vi "Generate Hologram.vi"(0 "x":sgl[](array[numeric]), 1 "y":sgl[](array[numeric]), 2 "z":sgl[](array[numeric]), 3 "spot_intensities":sgl[](array[numeric]) min=1, 4 "CUDA/SLM error in":errorcluster, 8 "path in":path, 9 "N_iterations":i32, 10 "method":i32, 12 "CGH in":u8[][](array[numeric])=array512x512[262144 elements]) -> (18 "path out":path, 20 "return":i32, 24 "CGH out":u8[][](array[numeric]), 25 "weights":sgl[][](graph)=[[0.32087266, 0.30867794, 0.31952837, 0.32111803, 0.32117248, 0.3210771, 0.32099402, 0.32094038, 0.32090643, 0.32088554], [0.32087216, 0.30864686, 0.31954217, 0.32109785, 0.3211845, 0.32108435, 0.32099703, 0.32094118, 0.3209064, 0.32088524], [0.32087475, 0.30863738, 0.3195775, 0.3210921, 0.32118624, 0.3210818, 0.32099742, 0.32094282, 0.32090908, 0.32088798], [0.3208743, 0.3086348, 0.31957102, 0.3210825, 0.3211723, 0.32108226, 0.32100248, 0.3209465, 0.3209109, 0.3208884], [0.32082918, 0.33360976, 0.32222247, 0.3205971, 0.32050273, 0.32060897, 0.32069725, 0.32075626, 0.3207928, 0.3208153], [0.3208285, 0.33361444, 0.32216293, 0.32054555, 0.32047704, 0.3205865, 0.32068458, 0.32074872, 0.32078892, 0.32081345], [0.3208247, 0.333552, 0.32235736, 0.32059258, 0.32051176, 0.32061282, 0.32069716, 0.32075158, 0.32078704, 0.3208098], [0.3208295, 0.33357766, 0.32223862, 0.32057458, 0.32048234, 0.32059732, 0.32069272, 0.3207548, 0.32079253, 0.3208156]], 27 "CUDA/SLM error out":errorcluster)   [LabVIEW 2012]
panel:
  out "Numeric":i32
  out "weights":sgl[](array[numeric])
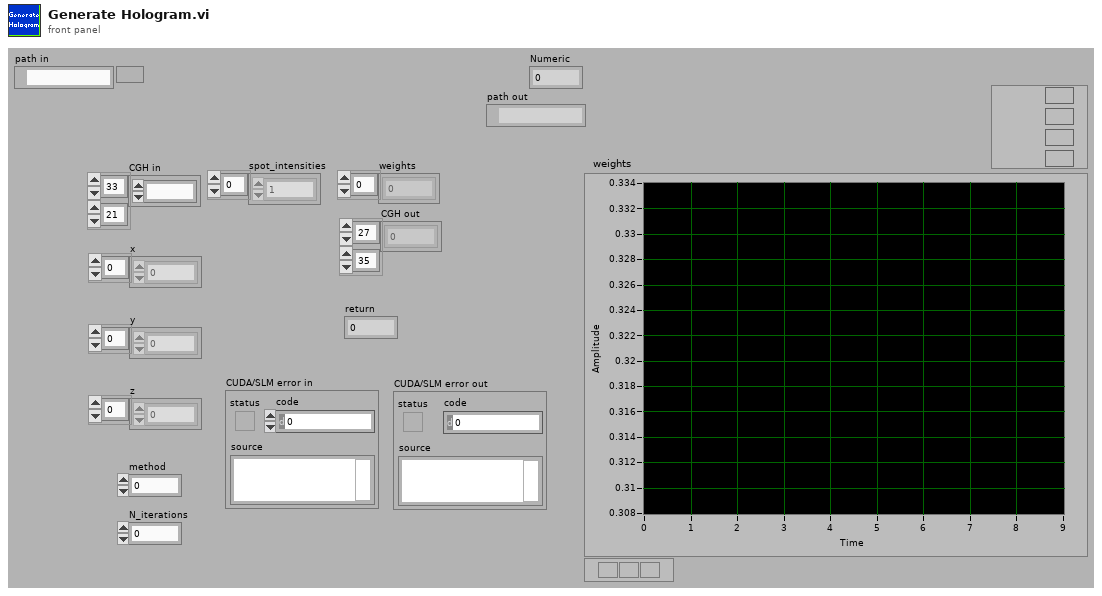
[diagram p1: front panel]
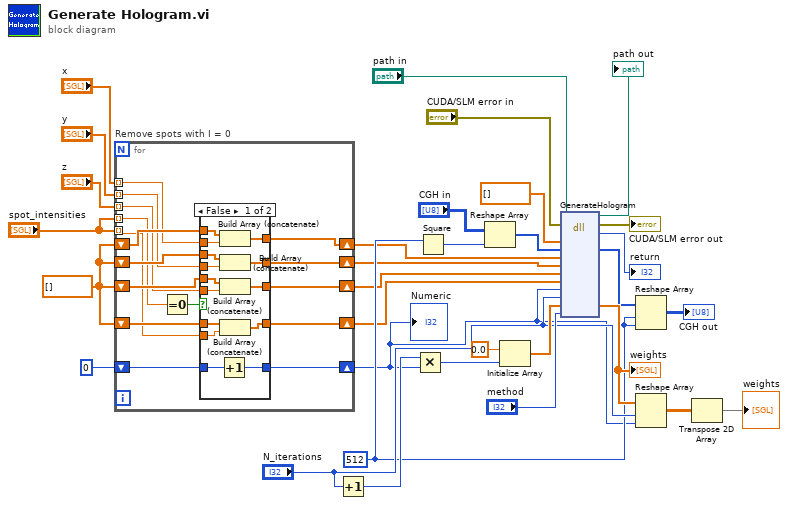
[diagram p0: block diagram]
diagram:
  w13 = sgl[] []
  w18 = 512 ("SLM size")
  n1 = for "Remove spots with I = 0" {
    shift-right: [w46] -> w6
    shift-left: w13 -> [w45]
    shift-right: [w44] -> w5
    shift-left: w13 -> [w43]
    shift-right: [w42] -> w4
    shift-left: w13 -> [w41]
    shift-right: [w47] -> w7
    shift-left: w13 -> [w40]
    shift-right: [w38] -> w3
    shift-left: 0 -> [w39]
    tunnel: "x" -> [w37] mode=indexing
    tunnel: "y" -> [w36] mode=indexing
    tunnel: "z" -> [w35] mode=indexing
    tunnel: "spot_intensities" -> [w34] mode=indexing
    tunnel: "spot_intensities" -> [w33] mode=indexing
    n2 = Equal To 0?(x=w33) -> (x = 0?=w48:bool)
    n3 = case shown="False" w48 {
      tunnel: w36 -> [w62 _]
      tunnel: w37 -> [w59 _]
      tunnel: [w53 w66] -> w47
      tunnel: [w61 w67] -> w46
      tunnel: w45 -> [w60 w67]
      tunnel: [w58 w65] -> w44
      tunnel: w43 -> [w57 w65]
      tunnel: [w56 w64] -> w42
      tunnel: w41 -> [w55 w64]
      tunnel: w40 -> [w54 w66]
      tunnel: [w52 w63] -> w38
      tunnel: w39 -> [w51 w63]
      tunnel: w35 -> [w50 _]
      tunnel: w34 -> [w49 _]
      frame False {
        n4 = Increment(x=w51) -> (x+1=w52:i32)
        n5 = Build Array (concatenate)(w54, w59) -> (w53:sgl[])
        n6 = Build Array (concatenate)(w60, w62) -> (w61:sgl[])
        n7 = Build Array (concatenate)(w57, w50) -> (w58:sgl[])
        n8 = Build Array (concatenate)(w55, w49) -> (w56:sgl[])
      }
      frame True {
      }
    }
  }
  "Numeric" <- w3
  n9 = Increment(x="N_iterations") -> (x+1=w28:i32)
  n10 = Multiply(x=w28, y=w3) -> (x*y=w27:i32)
  n11 = Square(x=w18) -> (x^2=w19:i32)
  n12 = Reshape Array("CGH in", w19) -> (w17:u8[])
  n13 = Initialize Array(sgl 0.0 ("element"), w27) -> (w25:sgl[])
  n14 = dll-call lib="D:/Dropbox/CUDA/GenerateHologramCUDA/C/x64/Release_PCIeSLM/GenerateHologramCUDA.dll" fn="GenerateHologram"(path in="path in", error in="CUDA/SLM error in", "V"=sgl[] [], "h_pSLM"=w17, "x"=w7, "y"=w6, "z"=w5, "spot_intensities"=w4, "N_spots"=w3, "N_iterations"="N_iterations", "weights"=w25, "method"="method") -> (path out=→"path out":path, error out=→"CUDA/SLM error out":errorcluster, "return"=→"return":i32, "h_pSLM"=w14:u8[], "weights"=w21:sgl[])  [unwired: 4 in, 5 out]
  "weights" <- w21
  n15 = Reshape Array(w14, w18, w18) -> (→"CGH out":u8[][])
  n16 = Reshape Array(w21, "N_iterations", w3) -> (w23:sgl[][])
  n17 = Transpose 2D Array(2D array=w23) -> (transposed array=→"weights":sgl[][])
